vi "GObjectFactory_FP.vi"(8 "error in":errorcluster, 11 "reference":refnum<vi>) -> (0 "error out":errorcluster, 3 "GObject out":refnum<class "GObject.lvclass">)   [LabVIEW 2014, in "GObject.lvclass"]
uses:
  GObject.lvclass
  Control/Control.lvclass
  Pane/Pane.lvclass
  Text/Text.lvclass
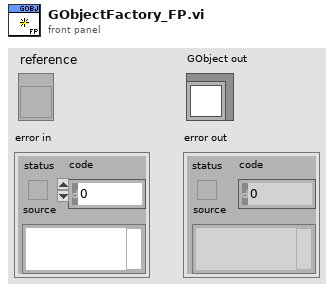
[diagram p1: front panel]
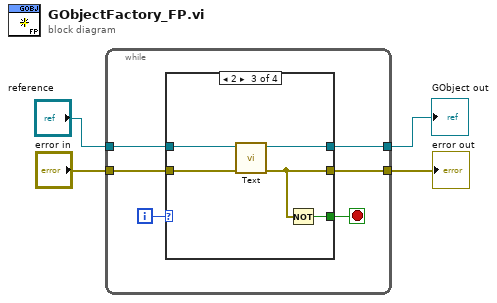
[diagram p0: block diagram]
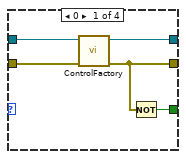
[diagram p2: hidden frame]
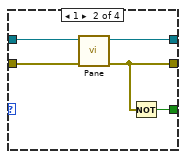
[diagram p3: hidden frame]
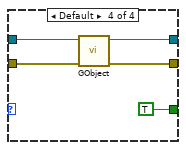
[diagram p4: hidden frame]
diagram:
  n1 = while {
    tunnel: "reference" -> [w9]
    tunnel: "error in" -> [w8]
    tunnel: [w7] -> w1
    tunnel: [w6] -> w2
    i -> [w10]
    stop <- w5 stop-if-true
    n2 = case shown="2" w10 {
      tunnel: w9 -> [w14 w19 w24 w28]
      tunnel: w8 -> [w15 w20 w25 w29]
      tunnel: [w11 w16 w21 w27] -> w7
      tunnel: [w13 w18 w23 w30] -> w6
      tunnel: [w12 w17 w22 TRUE] -> w5
      frame 0 {
        n3 = call "ControlFactory.vi"("error in"=w15, "Gen Refnum"=w14) -> ("error out"=w11:errorcluster, "Control out"=w13:refnum<class "Control.lvclass">)  [unwired: 8 in]
        n4 = Not(x=w11) -> (.not. x?=w12:bool)
      }
      frame 1 {
        n5 = call "Pane.vi"("error in"=w20, "Gen Refnum"=w19) -> ("error out"=w16:errorcluster, "Pane out"=w18:refnum<class "Pane.lvclass">)  [unwired: 8 in]
        n6 = Not(x=w16) -> (.not. x?=w17:bool)
      }
      frame 2 {
        n7 = call "Text.vi"("error in"=w25, "Gen Refnum"=w24) -> ("error out"=w21:errorcluster, "Text out"=w23:refnum<class "Text.lvclass">)  [unwired: 8 in]
        n8 = Not(x=w21) -> (.not. x?=w22:bool)
      }
      frame Default {
        n9 = call "GObject.vi"("error in"=w29, "reference"=w28) -> ("error out"=w27:errorcluster, "GObject out"=w30:refnum<class "GObject.lvclass">)  [unwired: 8 in]
      }
    }
  }
  "error out" <- w1
  "GObject out" <- w2
